vi "write-dbc-content.vi"(8 "error in (no error)":errorcluster, 10 "dbc.content":T1, 11 "dbc in":refnum<class "dbc.lvclass">) -> (0 "error out":errorcluster, 3 "dbc out":refnum<class "dbc.lvclass">)   [LabVIEW 2015, in "dbc.lvclass"]
uses:
  dbc.lvclass
  controls/dbc-content-data.ctl
  dbc.lvclass/dbc.ctl
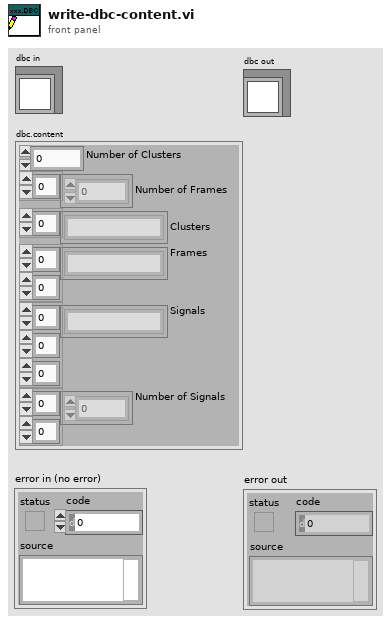
[diagram p1: front panel]
types:
  T1 = typedef "dbc-content-data.ctl" = cluster{"Number of Clusters":i32, "Number of Frames ":i32[], "Clusters":string[], "Frames":string[][], "Signals":string[][][], "Number of Signals":i32[][]}
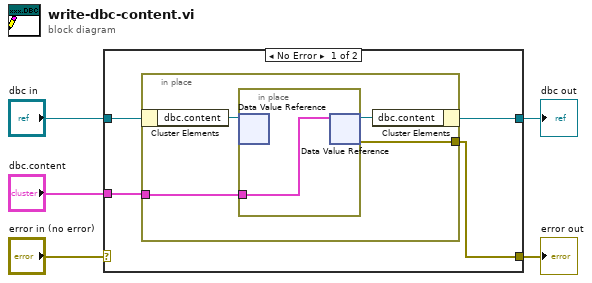
[diagram p0: block diagram]
diagram:
  n1 = case shown="No Error" "error in (no error)" {
    selector: "error in (no error)" -> [_ w15]
    tunnel: [w6 w15] -> w4
    tunnel: [w7 w16] -> w2
    tunnel: "dbc in" -> [w8 w16]
    tunnel: "dbc.content" -> [w9 _]
    frame No Error {
      n2 = in-place {
        in-place-border: [w11] -> w6
        in-place-border: w9 -> [w10]
        n3 = in-place-cluster #1(w8) -> ("dbc.content"=w13:refnum<data-value>)
        n4 = in-place {
          in-place-border: w10 -> [w14]
          n5 = in-place-dvr #2(w13) -> ()  [unwired: 2 out]
          n6 = in-place-dvr #2(w14) -> (w12:refnum<data-value>, w11:errorcluster)
        }
        n7 = in-place-cluster #1("dbc.content"=w12) -> (w7:refnum<class "dbc.lvclass">)
      }
    }
    frame Error {
    }
  }
  "error out" <- w4
  "dbc out" <- w2
